vi "Level Alert.vi"(4 "SensorCheck":T1, 6 "CtlRef":refnum<vi>, 7 "Event Common Data":cluster{"Source":T2, "Type":T3, "Time":u32} {"Source" items=["LabVIEW UI"=0, "ActiveX"=1, "User Event"=25]}) -> ()   [LabVIEW 2021]
uses:
  <vilib>/event_ctls.llb/eventsource.ctl
  <vilib>/event_ctls.llb/lveventtype.ctl
  tdefs/td.SensorCheck.ctl
  tdefs/td.Message.ctl
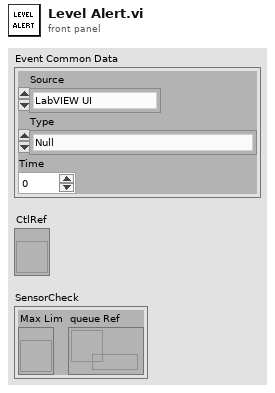
[diagram p1: front panel]
types:
  T1 = typedef "td.SensorCheck.ctl" = cluster{"Max Lim":refnum<vi>, "queue Ref":refnum<queue>}
  T2 = typedef "eventsource.ctl" = u32
  T3 = typedef "lveventtype.ctl" = enum32{"Null", "Timeout", "Annotation Menu Selection", "Annotation Menu Selection?", "App Instance Close", "App Instance Close?", "Autoscale Range Change", "Bookmark Info Change", "Cell Edit", "Cell Edit?", "Cursor Grab", "Cursor Grab?", "Cursor Menu Selection", "Cursor Menu Selection?", "Cursor Move", "Cursor Release", "Data Change", "Direction Change", "Display State Change", "Drag Ended", "Drag Enter", "Drag Leave", "Drag Over", "Drag Source Update", "Drag Starting", "Drag Starting?", "Drop", "Exec State Change", "Key Down", "Key Down?", "Key Repeat", "Key Repeat?", "Key Up", "Listbox Double Click", "Menu Activation?", "Menu Selection (App)", "Menu Selection? (App)", "Menu Selection (User)", "Mouse Down", "Mouse Down?", "Mouse Enter", "Mouse Leave", "Mouse Move", "Mouse Up", "Mouse Wheel", "NI Security User Change (App)", "Pane Size", "Panel Close", "Panel Close?", "Panel Resize", "Plot Attribute Change", "Scale Range Change", "Shortcut Menu Activation?", "Shortcut Menu Selection (App)", "Shortcut Menu Selection? (App)", "Shortcut Menu Selection (User)", "Tree Double Click", "Tree Drag", "Tree Drag?", "Tree Drop", "Tree Drop?", "Tree Item Close", "Tree Item Close?", "Tree Item Open", "Tree Item Open?", "User Event", "Value Change"}
  T4 = typedef "td.Message.ctl" = cluster{"Command":string, "Data":variant}
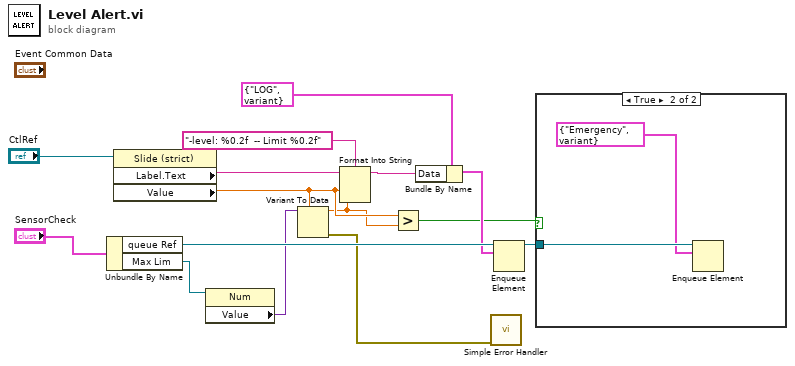
[diagram p0: block diagram]
diagram:
  n1 = Unbundle By Name("SensorCheck") -> ("queue Ref"=w14:refnum<queue>, "Max Lim"=w12:refnum<vi>)
  n2 = property class="Slide (strict)"(reference="CtlRef") -> ("Label.Text"=w10:string, "Value"=w4:dbl)  [unwired: 1 in, 2 out]
  n3 = property class="Num"(reference=w12) -> ("Value"=w8:variant)  [unwired: 1 in, 2 out]
  n4 = Variant To Data(type=w4, Variant=w8) -> (data=w3:dbl, error out=w7:errorcluster)  [unwired: 1 in]
  n5 = Format Into String(format string="-level: %0.2f  -- Limit %0.2f", initial string=w10, w4, w3) -> (resulting string=w5:string)  [unwired: 1 in, 1 out]
  n6 = Greater?(x=w4, y=w3) -> (0:w2:bool)
  n7 = Bundle By Name(cluster=T4 {"Command"="LOG", "Data"=variant} ("element"), "Data"=w5) -> (w6:T4)
  n8 = call <vilib>:"Simple Error Handler.vi"("error in (no error)"=w7) -> ()  [unwired: 4 in, 5 out]
  n9 = Enqueue Element(queue=w14, element=w6) -> (queue out=w1:refnum<queue>)  [unwired: 2 in, 2 out]
  n10 = case shown="True" w2 {
    tunnel: w1 -> [_ w17]
    frame False {
    }
    frame True {
      n11 = Enqueue Element(queue=w17, element=T4 {"Command"="Emergency", "Data"=variant}) -> ()  [unwired: 2 in, 3 out]
    }
  }
